vi "control_queues_release.vi"(8 "error in":errorcluster, 10 "Process names in":string[](array[string]), 11 "Process_communication in":variant) -> (0 "error out":errorcluster, 3 "Process_communication out":variant)   [LabVIEW 2011, in "Fiberscope_library.lvlib"]
uses:
  Fiberscope_library.lvlib
  typedefs/control_process_state_cluster.ctl
  typedefs/control_process_state_enum.ctl
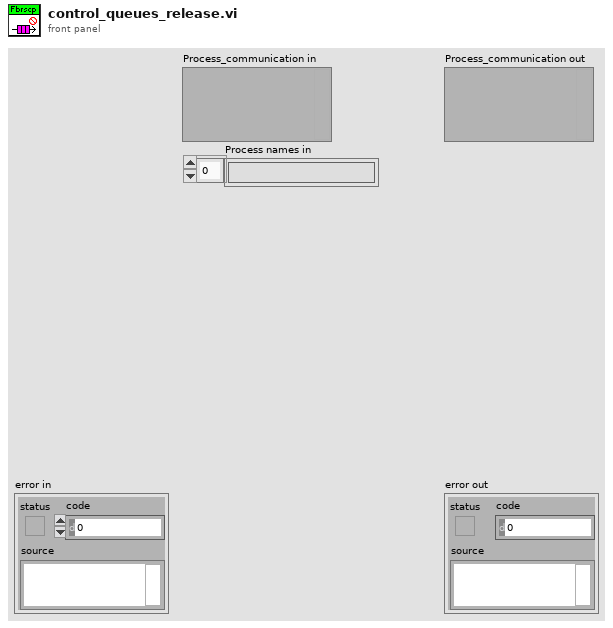
[diagram p1: front panel]
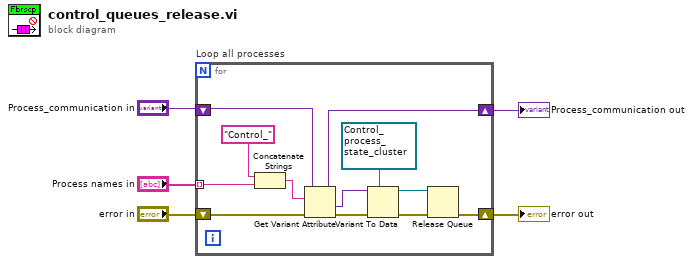
[diagram p0: block diagram]
diagram:
  n1 = for "Loop all processes" {
    shift-right: [w8] -> w4
    shift-left: "error in" -> [w14]
    tunnel: "Process names in" -> [w16] mode=indexing
    shift-right: [w12] -> w1
    shift-left: "Process_communication in" -> [w13]
    n2 = Concatenate Strings("Control_" ("string"), w16) -> (w15:string)
    n3 = Get Variant Attribute(Variant=w13, name=w15, error in=w14) -> (duplicate Variant=w12:variant, value=w10:variant, error out=w11:errorcluster)  [unwired: 1 in, 1 out]
    n4 = Variant To Data(error in=w11, type=refnum<queue> refnum ("queue out"), Variant=w10) -> (data=w6:refnum<queue>, error out=w7:errorcluster)
    n5 = Release Queue(queue=w6, error in (no error)=w7) -> (error out=w8:errorcluster)  [unwired: 1 in, 2 out]
  }
  "error out" <- w4
  "Process_communication out" <- w1
